vi "Module_p_control_sing_v2.vi"() -> ()   [LabVIEW 2014]
uses:
  <vilib>/eio/EIONode/EIONode.xnode
  <vilib>/rvi/eio/common/nirviEmuTemplateMethod_errors.vi
  <vilib>/rvi/FXPMathLib/FxpMul/XNode/nifxpmath_Multiplier.xnode
  <vilib>/rvi/FXPMathLib/sim/FxpSim.dll
  <vilib>/rvi/FXPMathLib/FxpSinAndCos/XNode/nifxpmath_SinAndCos.xnode
  <vilib>/rvi/FXPMathLib/FxpSinAndCos/simVIs/DllFxpSinAndCosTemp_sub.vi
  <vilib>/rvi/FXPMathLib/FxpSinAndCos/subVIs/nifxpmath_SinAndCos_SimConfig.ctl
  <vilib>/rvi/Analysis/measure/butterworth/XNode/niFpgaButterworthFilter.xnode
  <vilib>/rvi/FXPMathLib/FxpSub/XNode/nifxpmath_Sub.xnode
  <vilib>/rvi/FXPMathLib/FxpAdd/XNode/nifxpmath_Add.xnode
panel:
  out "Fp_PID":fxp<+/-,64,88>
  in  "viscois_cons_p":fxp<+/-,20,12>
  in  "fstp":fxp<+/-,20,12>
  in  "fcp":fxp<+/-,20,12>
  in  "Dp_d_tol":fxp<+,20,12>
  in  "fvp":fxp<+/-,20,12>
  in  "Friction tolorence_p":fxp<+/-,12,4>
  out "Friction comp_p":fxp<+/-,63,55> format="%.25g"
  in  "tolerance_Dp":fxp<+,64,87>
  out "Dpt_d":fxp<+/-,32,85>
  in  "Kd_p":fxp<+/-,16,1>
  out "Dp_tilde":fxp<+/-,64,74>
  in  "Kp_p":fxp<+/-,16,1>
  in  "coe_ini":bool
  out "Dpr":fxp<+/-,64,73>
  out "Dpr_ramp":fxp<+/-,64,73>
  out "Dpr_slope":fxp<+/-,62,41>
  in  "Dpr_time":fxp<+/-,41,11>
  in  "Dpr_end":fxp<+/-,20,10>
  in  "Ramp_start":bool
  out "Dpr_sin":fxp<+/-,35,5>
  in  "Sin_offset":fxp<+/-,34,4>
  in  "Sin_magnitude":fxp<+/-,17,2>
  out "Time now (s)":fxp<+,64,32>
  in  "Sin wave freq.(Hz)":fxp<+,1,2>=2.0
  in  "Dpr_sin/const":bool
  out "Dp_d":fxp<+/-,32,43>
  in  "Fmr":fxp<+/-,21,11>
  out "va_p":fxp<+/-,37,7>
  out "vb_p":fxp<+/-,38,8>
  out "vq_p_F":fxp<+/-,20,5> format="%.57g"
  out "vd_p_F":fxp<+/-,20,5>
  in  "Stop Motor_p":bool
  out "Dp_d(T method)":fxp<+/-,46,9>
  out "Omega_p(T)":fxp<+/-,20,9>
  in  "mt0_omega":u32
  out "mt_omaga":u32
  out "rad(NrTheta)_p":fxp<+/-,56,32>
  out "Dp(mm)":fxp<+/-,56,32>
  out "Encoder Position_p":i32
  in  "Encoder Reset_p":bool
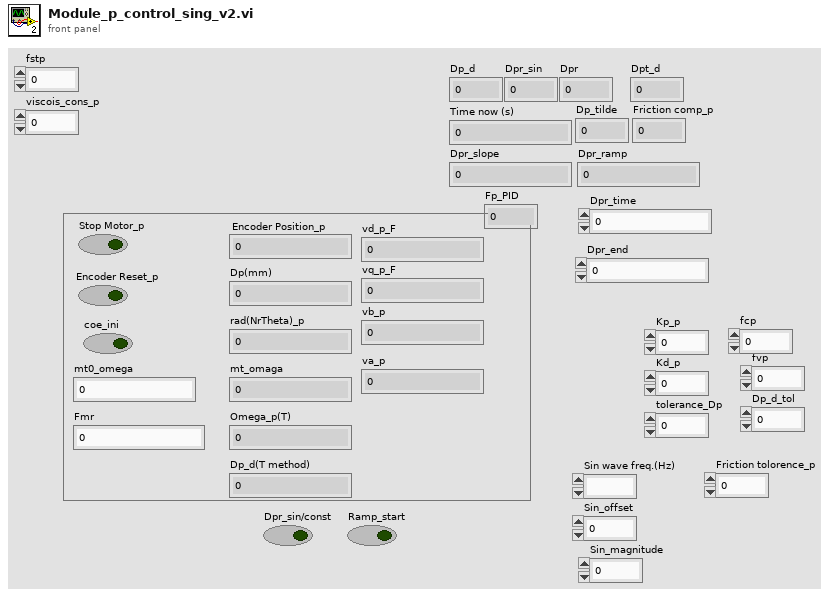
[diagram p1: front panel]
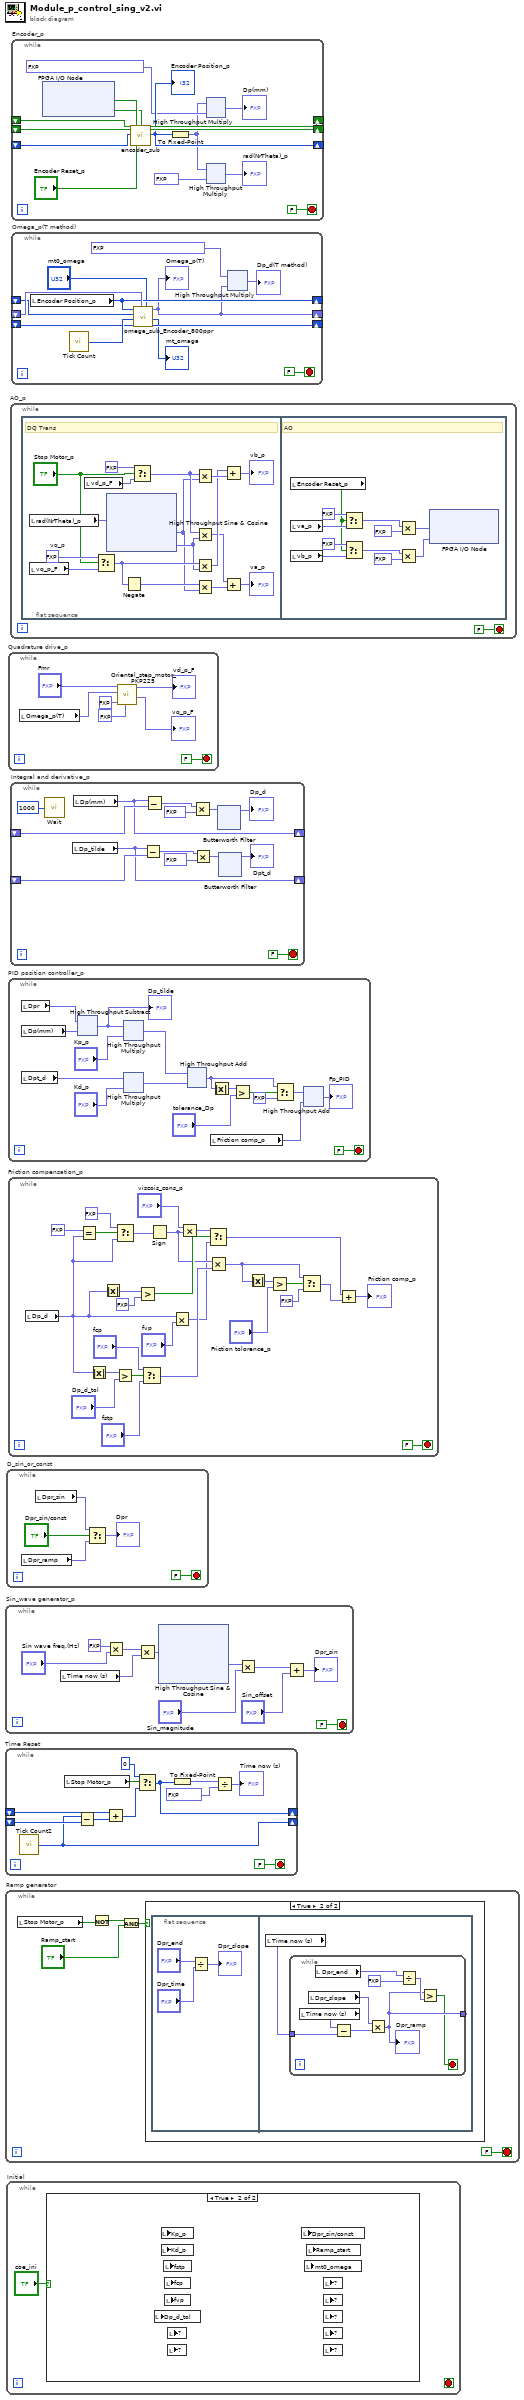
[diagram p0: block diagram]
diagram:
  n1 = while "Time Reset" {
    shift-right: [w5] -> _
    shift-left: _ -> [w9]
    shift-right: [w6] -> _
    shift-left: _ -> [w7]
    stop <- FALSE stop-if-true
    n2 = call "Tick Count2"() -> ("Tick Count(uSec)"=w6:u32)
    n3 = local read "Stop Motor_p"() -> (w12:bool)
    n4 = Subtract(x=w6, y=w7) -> (x-y=w8:u32)
    n5 = Add(x=w9, y=w8) -> (x+y=w10:u32)
    n6 = Select(t=u32 0, s=w12, f=w10) -> (s? t:f=w5:u32)
    n7 = To Fixed-Point(number=w5) -> (fixed-point=w2:fxp<+,32,32>)  [unwired: 1 in]
    n8 = Divide(x=w2, y=fxp<+,32,32> 1000000.0) -> (x/y=→"Time now (s)":fxp<+,64,32>)
  }
  n9 = while "Sin_wave generator_p" {
    stop <- FALSE stop-if-true
    n10 = local read "Time now (s)"() -> (w20:fxp<+,64,32>)
    n11 = Multiply(x=fxp<+,1,2> 2.0, y="Sin wave freq.(Hz)") -> (x*y=w21:fxp<+,1,3>)
    n12 = Multiply(x=w21, y=w20) -> (x*y=w19:fxp<+,64,34>)
    n13 = xnode "High Throughput Sine & Cosine"("x (pi)"=w19) -> ("sin(x)"=w18:fxp<+/-,17,2>)  [unwired: 1 out]
    n14 = Multiply(x=w18, y="Sin_magnitude") -> (x*y=w16:fxp<+/-,34,4>)
    n15 = Add(x=w16, y="Sin_offset") -> (x+y=→"Dpr_sin":fxp<+/-,35,5>)
  }
  n16 = while "Ramp generator" {
    stop <- FALSE stop-if-true
    n17 = local read "Stop Motor_p"() -> (w58:bool)
    n18 = Not(x=w58) -> (.not. x?=w57:bool)
    n19 = And(x=w57, y="Ramp_start") -> (x .and. y?=w55:bool)
    n20 = case shown="True" w55 {
      frame False {
      }
      frame True {
        n21 = flat-sequence {
          frame #0 {
            n22 = Divide(x="Dpr_end", y="Dpr_time") -> (x/y=→"Dpr_slope":fxp<+/-,62,41>)
          }
          frame #1 {
            n23 = local read "Time now (s)"() -> (w62:fxp<+,64,32>)
            n24 = while {
              tunnel: w62 -> [w70]
              tunnel: [w64] -> _
              stop <- w63 stop-if-true
              n25 = local read "Time now (s)"() -> (w71:fxp<+,64,32>)
              n26 = local read "Dpr_slope"() -> (w68:fxp<+/-,62,41>)
              n27 = local read "Dpr_end"() -> (w66:fxp<+/-,20,10>)
              n28 = Subtract(x=w71, y=w70) -> (x-y=w69:fxp<+/-,64,33>)
              n29 = Multiply(x=w68, y=w69) -> (x*y=w64:fxp<+/-,64,73>)
              "Dpr_ramp" <- w64
              n30 = Divide(x=w66, y=fxp<+,1,2> 2.0) -> (x/y=w65:fxp<+/-,21,9>)
              n31 = Greater?(x=w64, y=w65) -> (0:w63:bool)
            }
          }
        }
      }
    }
  }
  n32 = while "D_sin_or_const" {
    stop <- FALSE stop-if-true
    n33 = local read "Dpr_ramp"() -> (w74:fxp<+/-,64,73>)
    n34 = local read "Dpr_sin"() -> (w75:fxp<+/-,35,5>)
    n35 = Select(t=w75, s="Dpr_sin/const", f=w74) -> (s? t:f=→"Dpr":fxp<+/-,64,73>)
  }
  n36 = while "Initial" {
    stop <- _ stop-if-true
    n37 = case shown="True" "coe_ini" {
      frame False {
      }
      frame True {
        n38 = local read "Dp_d_tol"() -> ()  [unwired: 1 in]
        n39 = local read "Kp_p"() -> ()  [unwired: 1 in]
        n40 = local read "Kd_p"() -> ()  [unwired: 1 in]
        n41 = local read "fstp"() -> ()  [unwired: 1 in]
        n42 = local read "fcp"() -> ()  [unwired: 1 in]
        n43 = local read "fvp"() -> ()  [unwired: 1 in]
        n44 = local read item#-1() -> ()  [unwired: 1 in]
        n45 = local read item#-1() -> ()  [unwired: 1 in]
        n46 = local read "Dpr_sin/const"() -> ()  [unwired: 1 in]
        n47 = local read "mt0_omega"() -> ()  [unwired: 1 in]
        n48 = local read "Ramp_start"() -> ()  [unwired: 1 in]
        n49 = local read item#-1() -> ()  [unwired: 1 in]
        n50 = local read item#-1() -> ()  [unwired: 1 in]
        n51 = local read item#-1() -> ()  [unwired: 1 in]
        n52 = local read item#-1() -> ()  [unwired: 1 in]
        n53 = local read item#-1() -> ()  [unwired: 1 in]
      }
    }
  }
  n54 = while "Quadrature drive_p" {
    stop <- FALSE stop-if-true
    n55 = local read "Omega_p(T)"() -> (w79:fxp<+/-,20,9>)
    n56 = call "Oriental_step_motor_PKP225.vi"("F_Threshold"=fxp<+,12,12> 10.0, "dFmr"=fxp<+/-,25,15> 0.0, "omega"=w79, "Fmr"="Fmr") -> ("vq_F"=→"vq_p_F":fxp<+/-,20,5>, "vd_F"=→"vd_p_F":fxp<+/-,20,5>)  [unwired: 6 in]
  }
  n57 = while "PID position controller_p" {
    stop <- FALSE stop-if-true
    n58 = local read "Dpr"() -> (w100:fxp<+/-,64,73>)
    n59 = local read "Dp(mm)"() -> (w101:fxp<+/-,56,32>)
    n60 = local read "Dpt_d"() -> (w95:fxp<+/-,32,85>)
    n61 = xnode "High Throughput Subtract"("x"=w100, "y"=w101) -> ("x-y"=w99:fxp<+/-,64,74>)
    "Dp_tilde" <- w99
    n62 = xnode "High Throughput Multiply"("x"=w99, "y"="Kp_p") -> ("x*y"=w97:fxp<+/-,64,75>)
    n63 = xnode "High Throughput Multiply"("x"=w95, "y"="Kd_p") -> ("x*y"=w94:fxp<+/-,48,86>)
    n64 = xnode "High Throughput Add"("x"=w97, "y"=w94) -> ("x+y"=w90:fxp<+/-,64,87>)
    n65 = local read "Friction comp_p"() -> (w87:fxp<+/-,63,55>)
    n66 = Absolute Value(x=w90) -> (abs(x)=w93:fxp<+,64,87>)
    n67 = Greater?(x=w93, y="tolerance_Dp") -> (0:w91:bool)
    n68 = Select(t=w90, s=w91, f=fxp<+/-,64,87> 0.0) -> (s? t:f=w88:fxp<+/-,64,87>)
    n69 = xnode "High Throughput Add"("x"=w88, "y"=w87) -> ("x+y"=→"Fp_PID":fxp<+/-,64,88>)
  }
  n70 = while "Friction compensation_p" {
    stop <- FALSE stop-if-true
    n71 = local read "Dp_d"() -> (w106:fxp<+/-,32,43>)
    n72 = Equal?(x=fxp<+,1,1> 0.0 ("y"), y=w106) -> (x = y?=w116:bool)
    n73 = Absolute Value(x=w106) -> (abs(x)=w124:fxp<+,32,43>)
    n74 = Absolute Value(x=w106) -> (abs(x)=w118:fxp<+,32,43>)
    n75 = Select(t=fxp<+,20,10> 0.0, s=w116, f=w106) -> (s? t:f=w114:fxp<+/-,53,43>)
    n76 = Greater?(x=w124, y="Dp_d_tol") -> (0:w122:bool)
    n77 = Greater?(x=w118, y=fxp<+,20,12> 25.0) -> (0:w111:bool)
    n78 = Select(t="fcp", s=w122, f="fstp") -> (s? t:f=w119:fxp<+/-,20,12>)
    n79 = Sign(1:w114) -> (0:w110:fxp<+/-,2,2>)
    n80 = Multiply(x=w106, y="fvp") -> (x*y=w104:fxp<+/-,52,55>)
    n81 = Multiply(x="viscois_cons_p", y=w110) -> (x*y=w112:fxp<+/-,21,13>)
    n82 = Select(t=w112, s=w111, f=w104) -> (s? t:f=w108:fxp<+/-,63,55>)
    n83 = Multiply(x=w110, y=w119) -> (x*y=w103:fxp<+/-,21,13>)
    n84 = Absolute Value(x=w103) -> (abs(x)=w128:fxp<+,20,12>)
    n85 = Greater?(x=w128, y="Friction tolorence_p") -> (0:w129:bool)
    n86 = Select(t=w103, s=w129, f=fxp<+,20,12> 0.0) -> (s? t:f=w109:fxp<+/-,21,13>)
    n87 = Add(x=w108, y=w109) -> (x+y=→"Friction comp_p":fxp<+/-,63,55>)
  }
  n88 = while "AO_p" {
    stop <- FALSE stop-if-true
    n89 = flat-sequence {
      frame #0 {
        w147 = fxp<+,1,1> 0.0  # vq_p
        # "DQ Trans"
        n90 = local read "rad(NrTheta)_p"() -> (w140:fxp<+/-,56,32>)
        n91 = local read "vq_p_F"() -> (w146:fxp<+/-,20,5>)
        n92 = local read "vd_p_F"() -> (w141:fxp<+/-,20,5>)
        n93 = Select(t=w147, s="Stop Motor_p", f=w146) -> (s? t:f=w145:fxp<+/-,20,5>)
        n94 = xnode "High Throughput Sine & Cosine"("x (pi)"=w140) -> ("sin(x)"=w137:fxp<+/-,17,2>, "cos(x)"=w139:fxp<+/-,17,2>)
        n95 = Negate(x=w145) -> (-x=w144:fxp<+/-,21,6>)
        n96 = Select(t=fxp<+,1,1> 0.0, s="Stop Motor_p", f=w141) -> (s? t:f=w138:fxp<+/-,20,5>)
        n97 = Multiply(x=w138, y=w137) -> (x*y=w136:fxp<+/-,37,7>)
        n98 = Multiply(x=w138, y=w139) -> (x*y=w132:fxp<+/-,37,7>)
        n99 = Multiply(x=w145, y=w139) -> (x*y=w135:fxp<+/-,37,7>)
        n100 = Multiply(x=w144, y=w137) -> (x*y=w133:fxp<+/-,36,6>)
        n101 = Add(x=w135, y=w136) -> (x+y=→"vb_p":fxp<+/-,38,8>)
        n102 = Add(x=w132, y=w133) -> (x+y=→"va_p":fxp<+/-,37,7>)
      }
      frame #1 {
        # "AO"
        n103 = local read "Encoder Reset_p"() -> (w178:bool)
        n104 = local read "va_p"() -> (w180:fxp<+/-,37,7>)
        n105 = local read "vb_p"() -> (w179:fxp<+/-,38,8>)
        n106 = Select(t=fxp<+,2,2> 3.0, s=w178, f=w180) -> (s? t:f=w183:fxp<+/-,37,7>)
        n107 = Select(t=fxp<+,1,1> 0.0, s=w178, f=w179) -> (s? t:f=w184:fxp<+/-,38,8>)
        n108 = Multiply(x=w183, y=fxp<+/-,1,0> -0.5) -> (x*y=w188:fxp<+/-,37,6>)
        n109 = Multiply(x=w184, y=fxp<+/-,1,0> -0.5) -> (x*y=w187:fxp<+/-,37,6>)
        n110 = xnode "FPGA I/O Node"("Mod8/AO0"=w188, "Mod8/AO1"=w187) -> ()  [unwired: 2 in, 2 out]
      }
    }
  }
  n111 = while "Integral and derivative_p" {
    shift-right: [w197] -> _
    shift-left: _ -> [w198]
    shift-right: [w191] -> _
    shift-left: _ -> [w195]
    stop <- FALSE stop-if-true
    n112 = call "Wait"("Count(uSec)"=u32 1000) -> ()  [unwired: 1 out]
    n113 = local read "Dp_tilde"() -> (w191:fxp<+/-,64,74>)
    n114 = local read "Dp(mm)"() -> (w197:fxp<+/-,56,32>)
    n115 = Subtract(x=w191, y=w195) -> (x-y=w193:fxp<+/-,64,75>)
    n116 = Subtract(x=w197, y=w198) -> (x-y=w199:fxp<+/-,57,33>)
    n117 = Multiply(x=w199, y=fxp<+,7,10> 1000.0) -> (x*y=w201:fxp<+/-,64,43>)
    n118 = Multiply(x=w193, y=fxp<+,7,10> 1000.0) -> (x*y=w192:fxp<+/-,64,85>)
    n119 = xnode "Butterworth Filter"("input data"=w201) -> ("output data"=→"Dp_d":fxp<+/-,32,43>)  [unwired: 2 in]
    n120 = xnode "Butterworth Filter"("input data"=w192) -> ("output data"=→"Dpt_d":fxp<+/-,32,85>)  [unwired: 2 in]
  }
  n121 = while "Encoder_p" {
    shift-right: [w229] -> _
    shift-left: _ -> [w231]
    shift-right: [w228] -> _
    shift-left: _ -> [w230]
    shift-right: [w225] -> _
    shift-left: _ -> [w227]
    stop <- FALSE stop-if-true
    n122 = xnode "FPGA I/O Node"() -> ("Mod3/DIO0"=w233:bool, "Mod3/DIO1"=w232:bool)  [unwired: 2 in, 2 out]
    n123 = call "encoder_sub.vi"("A_pre"=w231, "B_pre"=w230, "Encoder Position_pre"=w227, "A input"=w233, "Encoder Position Reset"="Encoder Reset_p", "B input"=w232) -> ("A"=w229:bool, "B"=w228:bool, "Encoder Position (Counts)"=w225:i32)  [unwired: 19 in]
    "Encoder Position_p" <- w225
    n124 = To Fixed-Point(number=w225) -> (fixed-point=w222:fxp<+/-,32,32>)  [unwired: 1 in]
    n125 = xnode "High Throughput Multiply"("x"=w222, "y"=fxp<+/-,24,0> 0.002499997615814209) -> ("x*y"=→"Dp(mm)":fxp<+/-,56,32>)
    n126 = xnode "High Throughput Multiply"("x"=w222, "y"=fxp<+/-,24,0> 0.125) -> ("x*y"=→"rad(NrTheta)_p":fxp<+/-,56,32>)
  }
  n127 = while "Omega_p(T method)" {
    shift-right: [w243] -> _
    shift-left: _ -> [w244]
    shift-right: [w237] -> _
    shift-left: _ -> [w241]
    shift-right: [w239] -> _
    shift-left: _ -> [w240]
    stop <- FALSE stop-if-true
    n128 = local read "Encoder Position_p"() -> (w239:i32)
    n129 = call "Tick Count"() -> ("Tick Count(Ticks)"=w245:u32)
    n130 = call "omega_sub_Encoder_800ppr.vi"("mt0"="mt0_omega", "omega_pre"=w241, "ticks_m_pre"=w244, "ticks"=w245, "count_pre"=w240, "count"=w239) -> ("ticks_m"=w243:u32, "mt"=→"mt_omaga":u32, "omega"=w237:fxp<+/-,20,9>)  [unwired: 3 in]
    "Omega_p(T)" <- w237
    n131 = xnode "High Throughput Multiply"("x"=fxp<+/-,26,0> 0.3183099031448364, "y"=w237) -> ("x*y"=→"Dp_d(T method)":fxp<+/-,46,9>)
  }
